vi "Read ID.vi"(8 "error in (no error)":errorcluster, 11 "Channel in":refnum<class "Channel.lvclass">) -> (0 "error out":errorcluster, 2 "ID":u8, 3 "Channel out":refnum<class "Channel.lvclass">)   [LabVIEW 2018, in "Channel.lvclass"]
uses:
  Channel.lvclass
  Channel.lvclass/Channel.ctl
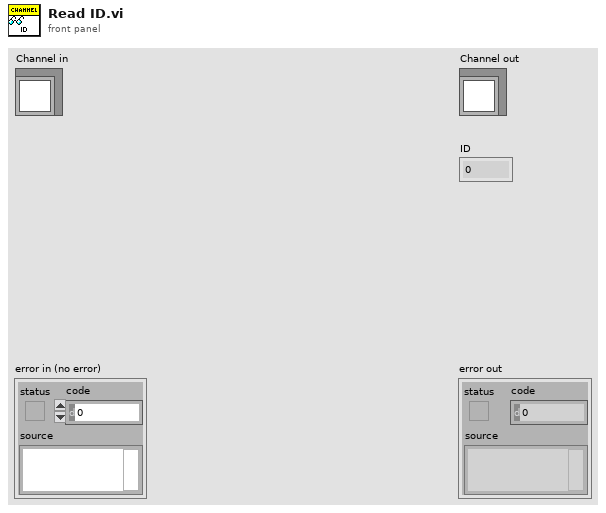
[diagram p1: front panel]
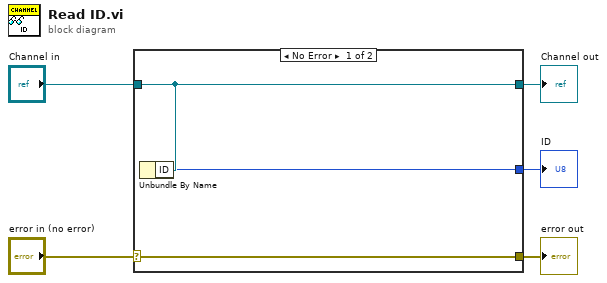
[diagram p0: block diagram]
diagram:
  n1 = case shown="No Error" "error in (no error)" {
    selector: "error in (no error)" -> [w8 w9]
    tunnel: [w8 w9] -> w4
    tunnel: [w7 w10] -> w2
    tunnel: "Channel in" -> [w7 w10]
    tunnel: [w6 _] -> w1
    frame No Error {
      n2 = Unbundle By Name(w7) -> ("ID"=w6:u8)
    }
    frame Error {
    }
  }
  "error out" <- w4
  "Channel out" <- w2
  "ID" <- w1
